vi "AlliGator Compute Phasor Plot for I-m-phi Dataset.vi"(6 "Harmonic index":i32, 8 "error in (no error)":errorcluster, 9 "Image Array":T1[](array[typedef]), 10 "Sum Image":T1, 11 "[[CSG]] Phasor Array in":csg[][](array[numeric])) -> (0 "error out":errorcluster, 1 "[[CSG]] Phasor Array out":csg[][](array[numeric]), 3 "Valid Pixel?":bool[][](array[boolean]))   [LabVIEW 2021, in "AlliGator Phasor Plot.lvlib"]
doc: "Computes the Phasor Plot for a FLIMBox dataset."
uses:
  AlliGator Phasor Plot.lvlib
  <vilib>/vision/Image Controls.llb/IMAQ Image.ctl
  Settings/AlliGator Pixel Counts Constraints.ctl
  Settings/AlliGator High Count Pixels Rejection Options.ctl
  Settings/AlliGator Low Count Pixels Rejection Options.ctl
  Globals, Variables, Constants/AlliGator Variables List.ctl
  Globals, Variables, Constants/AlliGator Globals, Variables & Constants.lvlib
  Settings/AlliGator Settings.lvlib
  Source Image/AlliGator Source Image.lvlib
  Arrays/Arrays.lvlib
  Utilities/Utilities.lvlib
panel:
  out "Same size arrays":bool
  # "see the AlliGator License on the block diagram (Ctrl+E or Window:Show Block Diagram)"
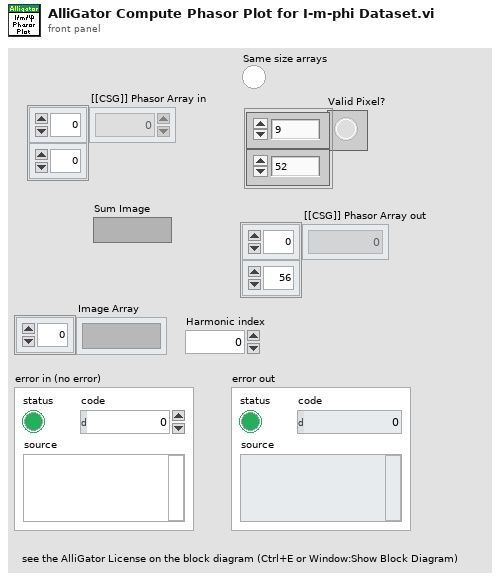
[diagram p1: front panel]
types:
  T1 = typedef "IMAQ Image.ctl" = refnum<image>
  T2 = typedef "AlliGator Settings.lvlib/AlliGator Pixel Counts Constraints.ctl" = cluster{"High Count Pixels Rejection Options":T3, "Low Count Pixels Rejection Options":T4}
  T3 = typedef "AlliGator Settings.lvlib/AlliGator High Count Pixels Rejection Options.ctl" = cluster{"Background High Threshold Factor":dbl, "Fixed High Background Threshold":dbl, "Reject High Count Pixels":bool, "High Percentile":dbl}
  T4 = typedef "AlliGator Settings.lvlib/AlliGator Low Count Pixels Rejection Options.ctl" = cluster{"Background Low Threshold Factor":dbl, "Fixed Low Background Threshold":dbl, "Reject Low Count Pixels":bool, "Low Percentile":dbl}
  T5 = typedef "AlliGator Globals, Variables & Constants.lvlib/AlliGator Variables List.ctl" = enum16{"---- GUI ----", "GUI:Initialization Status", "GUI:State Indicators Refnum", "GUI:Original AlliGator Menu Items", "GUI:Current Action Loop State", "GUI:Script in progress", "GUI:Playback", "GUI:Loop Playback", "GUI:Search ROI Used", "GUI:Search ROI", "Decay Graph Max Legend Size", "Intensity Graph Max Legend Size", "Decay Statistics Graph Max Legend Size", "Phasor Graph Max Legend Size", "Phasor Ratio Graph Max Legend Size", "Lifetime Graph Max Legend Size", "---- Files ----", "Files:Export Dataset Frames as Individual Files", "Files:Show Batch Export Help Balloons", "Files:Frames in Dataset", "Files:ptu File Frame Start Indices", "Files:Current Frame in Dataset", "Files:Current Frame Timestamp", "Files:Dataset Loaded", "Files:Dataset Metadata", "Files:Dataset Channel", "Files:Dataset Data Description", "Files:Background Dataset Metadata", "Files:Background Dataset Channel", "Files:Background Dataset Data Description", "Files:Background File Subtraction", "Files:Background File Path", "Files:Background File Pile-up Correction", "Files:Background File Pixel Well Capacity", "Files:Background File Scaling Factor", "Files:Current Dataset Load Settings", "Files:Dataset Path", "Files:ICCD-specific Information", "Files:Macrotime Gate Separation", "------ Python Plugins ------", "Python Plugins:Information", "Python Plugins:Python Session", "Python Plugins:Valid Python Session?", "---- Source Image ----", "Source Image:ROIs", "Source Image:Current ROI", "Source Image:ROI Event Refnum", "X_Source Image Display Range", "X_Source Image Palette Information", "X_Type of Displayed Image", "X_Time Gate Slider", "Source Image:Palette List", "Source Image:Scale", "Source Image:ROI Overlay Color", "Source Image:Overlay to Erase", "Source Image:Is Displayed Image Accumulated", "Source Image:White Light Image Modified", "Source Image:Mask Image Modified", "---- Image Profile Window ----", "Image Profile:Window Event Refnum", "Image Profile:IntensityType", "Image Profile:Intensity Average Type", "Image Profile:Intensity-weighted SDV", "Image Profile:Box Profile Type", "Image Profile:Window Open", "Image Profile:Plotted Fit Parameter", "------ Phasor Graph -------", "Phasor Graph:Show Line", "---- Phasor Plot ---", "Phasor Plot:Parameters Changed", "Phasor Plot:FLI Dataset Modified since last Calculation", "Phasor Harmonics Data", "Selected Phasor Harmonics", "Phasor Harmonic Manager Event Refnum", "Phasor Plot:ROIs", "Phasor Plot:Current ROI", "Phasor Plot:ROI Event Refnum", "Phasor Plot:Image Reference Points", "Phasor Plot:Computed", "Phasor Plot:Palette Information", "Phasor Plot:Palette List", "Phasor Plot:Phasor Ratio Palette Information", "Phasor Plot:Phasor Ratio Palette List", "Phasor Plot:Image Scale", "Phasor Plot:Image Overlay to Erase", "Phasor Plot:Image Elements to Update", "Phasor Plot:Current Calculation Parameters", "Phasor Plot:Current Calibration Options", "Phasor Plot:Reset Cumulated Phasor Plot", "Phasor Plot:Reference 1", "Phasor Plot:Lifetime Reference 1", "Phasor Plot:Reference 1 Frequency", "Phasor Plot:Reference 2", "Phasor Plot:Lifetime Reference 2", "Phasor Plot:Reference 2 Frequency", "---- Decay Analysis ----", "Number of Selected Decays to Fit", "LS Fit Results", "LAR Fit Results", "BS Fit Results", "Last Decay Max - Min", "Best Fit Parameters", "Best Fit Parameter Names", "Actual Size X", "Actual Size Y", "Binning X", "Binning Y", "Actual # Gates", "Dataset Number", "Gates to...", "Gates Skipped", "Gates to keep", "Gate Step", "Gate Separation", "Reversed Gates", "Pile-up Correction", "Pixel Well Capacity", "Background Subtracted", "Background Subtraction Method", "Background Definition Range", "Background File (deprecated)", "Number of Dataset Accumulated", "Array of Accumulated Dataset Paths", "Do Averaged Datasets", "Destination File Path", "Process Plot Target", "Use 1/D as Phasor Frequency", "---- Decay Fit Parameter Map -----", "Decay Fit Parameter Map:Palette Information", "Decay Fit Parameter Map:Palette List", "---- Parameter Map ----", "Parameter Map:Palette Information", "Parameter Map:Palette List", "------- Local Decay Window ---------", "Local Decay Graph Window:Event Refnum", "Local Decay Graph Window:Use normalized IRF for convolution", "----- Miscellaneous ----", "Misc:Skippable Dialog Windows Status"}
  T6 = typedef "AlliGator Phasor Plot.lvlib/AlliGator Phasor Plot Parameters v2.ctl" = cluster{"Phasor Frequency":dbl[unit], "Decay Preprocessing Options & Parameters":T7, "FLI Dataset Modified":bool, "Source Image Settings":cluster{"Low Count Pixels Rejection Options":T4, "High Count Pixels Rejection Options":T3}, "Data Information":cluster{"Gate Width":dbl[unit], "Gate Separation":dbl[unit], "Step (Gate Separation)":i32, "Laser Period":dbl[unit], "SYNC Period":dbl[unit], "Channel Name":u16, "Channel Arithmetic":T13, "Pile-up Correction":bool, "Pixel Well Capacity":u32, "Dataset Scaling Factor":dbl}, "Phasor Plot":cluster{"Phasor Plot Smoothing Options":T14, "Phasor Plot Size":T17, "Selected Image ROI(s)":bool, "All Image ROIs":bool, "Selected Source Image ROI":i32, "Source Image ROIs":T18[]}}
  T7 = typedef "AlliGator Decay Analysis.lvlib/AlliGator Decay Preprocessing.lvlib/AlliGator Decay Preprocessing Options.ctl" = cluster{"Background Subtraction Parameters":T8, "Decay Preprocessing Parameters":T10, "Preprocessing Steps Order":string[]}
  T8 = typedef "AlliGator Decay Analysis.lvlib/AlliGator Decay Preprocessing.lvlib/AlliGator Background Subtraction Parameters.ctl" = cluster{"Background Definition Range":cluster{"Min Gate":dbl[unit], "Max Gate":dbl[unit]}, "Baseline Subtraction Method":T9, "Background Subtraction?":bool, "Background File":path, "Background Constant":dbl, "Background Scaling Factor":dbl, "Background Pile-up Correction":bool, "Background Pixel Well Capacity":u32}
  T9 = typedef "AlliGator Decay Analysis.lvlib/AlliGator Decay Preprocessing.lvlib/AlliGator Baseline Subtraction Method.ctl" = enum16{"Mean", "Min", "Square Gated Single-Exponential", "File", "Constant"}
  T10 = typedef "AlliGator Decay Analysis.lvlib/AlliGator Decay Preprocessing.lvlib/AlliGator Decay Preprocessing Parameters.ctl" = cluster{"Background Subtraction":bool, "Straighten Decay":bool, "Reverse Gates":bool, "1-Normalized Decay":bool, "Smoothen Decay":bool, "Smoothing Parameter":dbl, "Shift Decay":bool, "Decay Shift Parameters":T11, "Extrapolate Decay":bool, "Additional Points":u32, "Head Fraction":dbl, "Pixel-Normalize Decay":bool, "Use Periodicity":bool, "Use Cursors":bool, "Tail Fraction":dbl, "Use Decay Pre-Processing":bool, "Fold Decay":bool, "# Folds":u32, "[0-1]-Normalized Decay":bool}
  T11 = typedef "XY Graph Add-Ons.lvlib/XY Graph Plot Shift Parameters.ctl" = cluster{"Type":T12, "Shift":dbl[unit], "Threshold":dbl, "Rotate":bool}
  T12 = typedef "XY Graph Add-Ons.lvlib/XY Graph Plot Shift Method.ctl" = enum16{"Default", "CFD", "Threshold", "Cross-Correlation"}
  T13 = typedef "AlliGator Settings.lvlib/AlliGator Gate Arithmetic.ctl" = enum16{"None", "INT-G2", "G2/INT*<INT>", "(1 - G2/INT)*<INT>"}
  T14 = typedef "AlliGator Phasor Plot.lvlib/AlliGator Phasor Plot Smoothing Options.ctl" = cluster{"Use Phasor Plot Smoothing":bool, "Kernel Type":T15, "Bin":i32, "Algorithm":T16}
  T15 = typedef "Arrays.lvlib/Kernel Type.ctl" = enum16{"Uniform", "Bilinear", "Gaussian"}
  T16 = typedef "Arrays.lvlib/Smoothing Algorithm.ctl" = enum16{"Rapid", "Thorough"}
  T17 = typedef "AlliGator Phasor Plot.lvlib/AlliGator Phasor Plot Size.ctl" = cluster{"H":i32, "V":i32, "Margin":dbl}
  T18 = typedef "Image.lvlib/Named ROI Description.ctl" = cluster{"ROI Descriptor":T19, "ROI Name":string, "Overlay Color":u32}
  T19 = typedef "ROI Descriptor" = cluster{"Global Rectangle":i32[], "Contours":cluster{"ID":enum32{"External", "Internal"}, "Type":u32, "Coordinates":i32[]}[]}
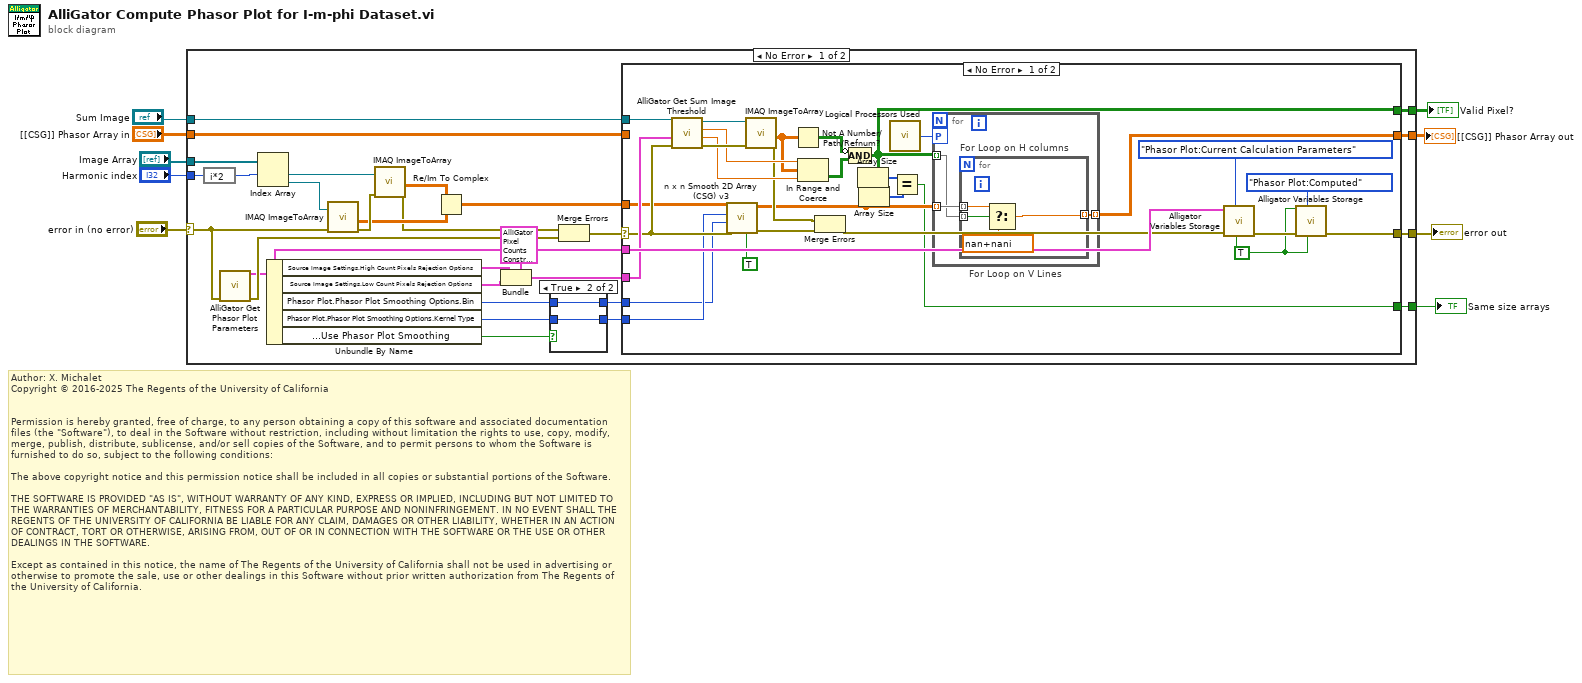
[diagram p0: block diagram]
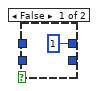
[diagram p2: hidden frame]
diagram:
  # "Author: X. Michalet\nCopyright © 2016-2025 The Regents of the University of California\n \n\nPermission is hereby granted, free of charge, to any person obtaining a copy of this software and associated documentation files (the \"Software\"), to deal in the Software without restriction, including without limitation the rights to use, copy, modify, merge, publish, distribute, sublicense, and/or sell copies of the Software, and to permit persons to whom the Software is furnished to do so, subject to the following conditions:\n\nThe above copyright notice and this permission notice shall be included in all copies or substantial portions of the Software.\n\nTHE SOFTWARE IS PROVIDED \"AS IS\", WITHOUT WARRANTY OF ANY KIND, EXPRESS OR IMPLIED, INCLUDING BUT NOT LIMITED TO THE WARRANTIES OF MERCHANTABILITY, FITNESS FOR A PARTICULAR PURPOSE AND NONINFRINGEMENT. IN NO EVENT SHALL THE REGENTS OF THE UNIVERSITY OF CALIFORNIA BE LIABLE FOR ANY CLAIM, DAMAGES OR OTHER LIABILITY, WHETHER IN AN ACTION OF CONTRACT, TORT OR OTHERWISE, ARISING FROM, OUT OF OR IN CONNECTION WITH THE SOFTWARE OR THE USE OR OTHER DEALINGS IN THE SOFTWARE.\n\nExcept as contained in this notice, the name of The Regents of the University of California shall not be used in advertising or otherwise to promote the sale, use or other dealings in this Software without prior written authorization from The Regents of the University of California."
  n1 = case shown="No Error" "error in (no error)" {
    selector: "error in (no error)" -> [w24 w81]
    tunnel: "Image Array" -> [w38 _]
    tunnel: "Harmonic index" -> [w33 _]
    tunnel: [w28 w82] -> w6
    tunnel: [w26 w81] -> w5
    tunnel: "[[CSG]] Phasor Array in" -> [w29 w82]
    tunnel: "Sum Image" -> [w25 _]
    tunnel: [w11 _] -> w2
    tunnel: [w10 _] -> w1
    frame No Error {
      n2 = expression code="i*2"(w33) -> (w37:i32)
      n3 = call "AlliGator Get Phasor Plot Parameters.vi"("Error In"=w24) -> ("Error Out"=w16:errorcluster, "Phasor Plot Parameters"=w12:T6)  [unwired: 8 in, 1 out]
      n4 = Index Array(array=w38, index #1=w37) -> (element #1=w36:T1, element #2=w35:T1)  [unwired: 1 in]
      n5 = Unbundle By Name(w12) -> ("Source Image Settings.High Count Pixels Rejection Options"=w22:T3, "Source Image Settings.Low Count Pixels Rejection Options"=w21:T4, "Phasor Plot.Phasor Plot Smoothing Options.Bin"=w20:i32, "Phasor Plot.Phasor Plot Smoothing Options.Kernel Type"=w19:T15, "Phasor Plot.Phasor Plot Smoothing Options.Use Phasor Plot Smoothing"=w18:bool)
      n6 = call "IMAQ ImageToArray"("error in (no error)"=w24, "Image"=w35) -> ("Image Pixels (Float)"=w31:sgl[][], "error out"=w34:errorcluster)  [unwired: 2 in, 3 out]
      n7 = call "IMAQ ImageToArray"("error in (no error)"=w34, "Image"=w36) -> ("Image Pixels (Float)"=w32:sgl[][], "error out"=w30:errorcluster)  [unwired: 2 in, 3 out]
      n8 = Re/Im To Complex(1:w31, 2:w32) -> (0:w27:csg[][])
      n9 = Bundle(cluster=T2 {"High Count Pixels Rejection Options"={"Background High Threshold Factor"=0.0, "Fixed High Background Threshold"=0.0, "Reject High Count Pixels"=FALSE, "High Percentile"=0.0}, "Low Count Pixels Rejection Options"={"Background Low Threshold Factor"=0.0, "Fixed Low Background Threshold"=0.0, "Reject Low Count Pixels"=FALSE, "Low Percentile"=0.0}} ("Pixel Counts Constraints"), "High Count Pixels Rejection Options"=w22, "Low Count Pixels Rejection Options"=w21) -> (w15:T2)
      n10 = case shown="True" w18 {
        tunnel: w20 -> [_ w41]
        tunnel: w19 -> [_ w40]
        tunnel: [1 ("Bin") w41] -> w13
        tunnel: [_ w40] -> w14
        frame False {
        }
        frame True {
        }
      }
      n11 = Merge Errors(w30, w16) -> (w17:errorcluster)
      n12 = case shown="No Error" w17 {
        selector: w17 -> [w57 w79]
        tunnel: w29 -> [_ w80]
        tunnel: [w53 w80] -> w28
        tunnel: w27 -> [w54 _]
        tunnel: [w67 w79] -> w26
        tunnel: w25 -> [w64 _]
        tunnel: w15 -> [w63 _]
        tunnel: w14 -> [w56 _]
        tunnel: w13 -> [w55 _]
        tunnel: w12 -> [w66 _]
        tunnel: [w48 _] -> w11
        tunnel: [w43 _] -> w10
        frame No Error {
          w70 = TRUE ("Get(F)/Set")
          n13 = call "AlliGator Get Sum Image Threshold.vi"("error in (no error)"=w57, "Pixel Counts Constraints"=w63, "Image in"=w64) -> ("error out"=w61:errorcluster, "Pixel Threshold Low"=w59:sgl, "Pixel Threshold High"=w60:sgl, "Image out (dup)"=w62:T1)  [unwired: 2 in, 3 out]
          n14 = call "n x n Smooth 2D Array (CSG) v3.vi"("Average"=TRUE, "Error In"=w57, "Kernel Size"=w55, "Kernel Type"=w56, "Array in"=w54) -> ("Error Out"=w52:errorcluster, "Array out"=w47:csg[][])  [unwired: 4 in, 1 out]
          n15 = call "IMAQ ImageToArray"("error in (no error)"=w61, "Image"=w62) -> ("Image Pixels (Float)"=w58:sgl[][], "error out"=w51:errorcluster)  [unwired: 2 in, 3 out]
          n16 = Not A Number/Path/Refnum?(number/path/refnum=w58) -> (NaN/Path/Refnum?=w65:bool[][])
          n17 = In Range and Coerce(upper limit=w60, x=w58, lower limit=w59) -> (In Range?=w44:bool[][])  [unwired: 1 out]
          n18 = Merge Errors(w51, w52) -> (w50:errorcluster)
          n19 = Compound Arithmetic op=AND(invert w65, w44) -> (w48:bool[][])
          n20 = Array Size(array=w48) -> (size(s)=w46:i32[])
          n21 = Array Size(array=w47) -> (size(s)=w45:i32[])
          n22 = call "Logical Processors Used.vi"() -> ("# Logical Processor Used"=w42:i32)  [unwired: 6 in]
          n23 = Equal?(x=w46, y=w45) -> (x = y?=w43:bool)
          n24 = for "For Loop on V Lines" {
            tunnel: w48 -> [w72] mode=indexing
            tunnel: w47 -> [w74] mode=indexing
            tunnel: [w73] -> w53 mode=indexing
            workers-P: w42 -> [_]
            n25 = for "For Loop on H columns" {
              tunnel: w74 -> [w78] mode=indexing
              tunnel: [w76] -> w73 mode=indexing
              tunnel: w72 -> [w75] mode=indexing
              n26 = Select(t=w78, s=w75, f=csg nan+nani) -> (s? t:f=w76:csg)
            }
          }
          n27 = call "Alligator Variables Storage.vi"("Get(F)/Set"=w70, "AlliGator Variable"=AlliGator_Variables_List."Phasor Plot:Current Calculation Parameters" ("Alligator Variable"), "Error In"=w50, "Data in"=w66) -> ("Error Out"=w71:errorcluster)  [unwired: 5 in, 2 out]
          n28 = call "Alligator Variables Storage.vi"("Get(F)/Set"=w70, "AlliGator Variable"=AlliGator_Variables_List."Phasor Plot:Computed" ("Alligator Variable"), "Error In"=w71, "Data in"=w70) -> ("Error Out"=w67:errorcluster)  [unwired: 5 in, 2 out]
        }
        frame Error {
        }
      }
    }
    frame Error {
    }
  }
  "[[CSG]] Phasor Array out" <- w6
  "error out" <- w5
  "Valid Pixel?" <- w2
  "Same size arrays" <- w1
